vi "testaCorrente+PSuc.vi"() -> ()   [LabVIEW 2019]
uses:
  <vilib>/DAQmx/write.llb/DAQmx Write (Digital Bool 1Line 1Point).vi
  <vilib>/Analysis/5stat.llb/RMS (DBL).vi
  <vilib>/DAQmx/write.llb/DAQmx Write (Counter Frequency 1Chan 1Samp).vi
  <vilib>/DAQmx/create/channels.llb/DAQmx Create Channel (DO-Digital Output).vi
  <vilib>/DAQmx/miscellaneous.llb/DAQmx Fill In Error Info.vi
  <vilib>/DAQmx/create/channels.llb/DAQmx Create Channel (CO-Pulse Generation-Frequency).vi
  <vilib>/DAQmx/configure/timing.llb/DAQmx Timing (Implicit).vi
  <resource>/objmgr/daqmx.rc
  <vilib>/Analysis/NI_AALPro.lvlib
  <vilib>/Analysis/NI_AALBase.lvlib
panel:
  out "Array":sgl[](array[numeric])
  out "Numeric":dbl
  out "Reading":bool=TRUE
  in  "STOP":bool
  out "Erro Corrente":errorcluster
  in  "Tab Control":T1(tab)
  out "GE Comp S [bar]":dbl
  out "GE Valv S [bar]":dbl
  out "Grafico Pressão":T2(graph)
  in  "Ativar Ventilador?":bool=TRUE
  out "Descarga [bar]":dbl
  out "Sucção [bar]":dbl
  out "Corrente RMS [A]":dbl
  out "Grafico Corrente":dbl(graph)
  out "Posição Atual da Válvula de Descarga":dbl format="%#_9f"
  out "Intermed [bar]":dbl
  in  "Frequência PWM [Hz]":dbl=2.0 min=1e-12
  out "G Pressão de Descarga":cluster{"Descarga [bar]":dbl}(graph)
  out "G Pressão de Sucção":cluster{"Sucção [bar]":dbl}(graph)
  out "G Corrente RMS":dbl(graph)
  out "G Pressão Intermed":dbl(graph)
  out "Error Out":errorcluster
  in  "Limpar Gráficos":bool
  out "Tempo de Ensaio":string
  in  "Ativar Compressor?":bool
  out "Erro Valv. Sucção":errorcluster
  out "Erro Pressão":errorcluster
  # "Pressão"
  # "Temperatura"
  # "Corrente"
  # "Vazão"
  # "Vibração"
  # "Controle Manual"
  # "Controle Aplicado"
  # "PID"
  # "Ranges"
  # "Arquivos"
  # "Resistência"
  # "Identificação de sistemas"
  # "Erros"
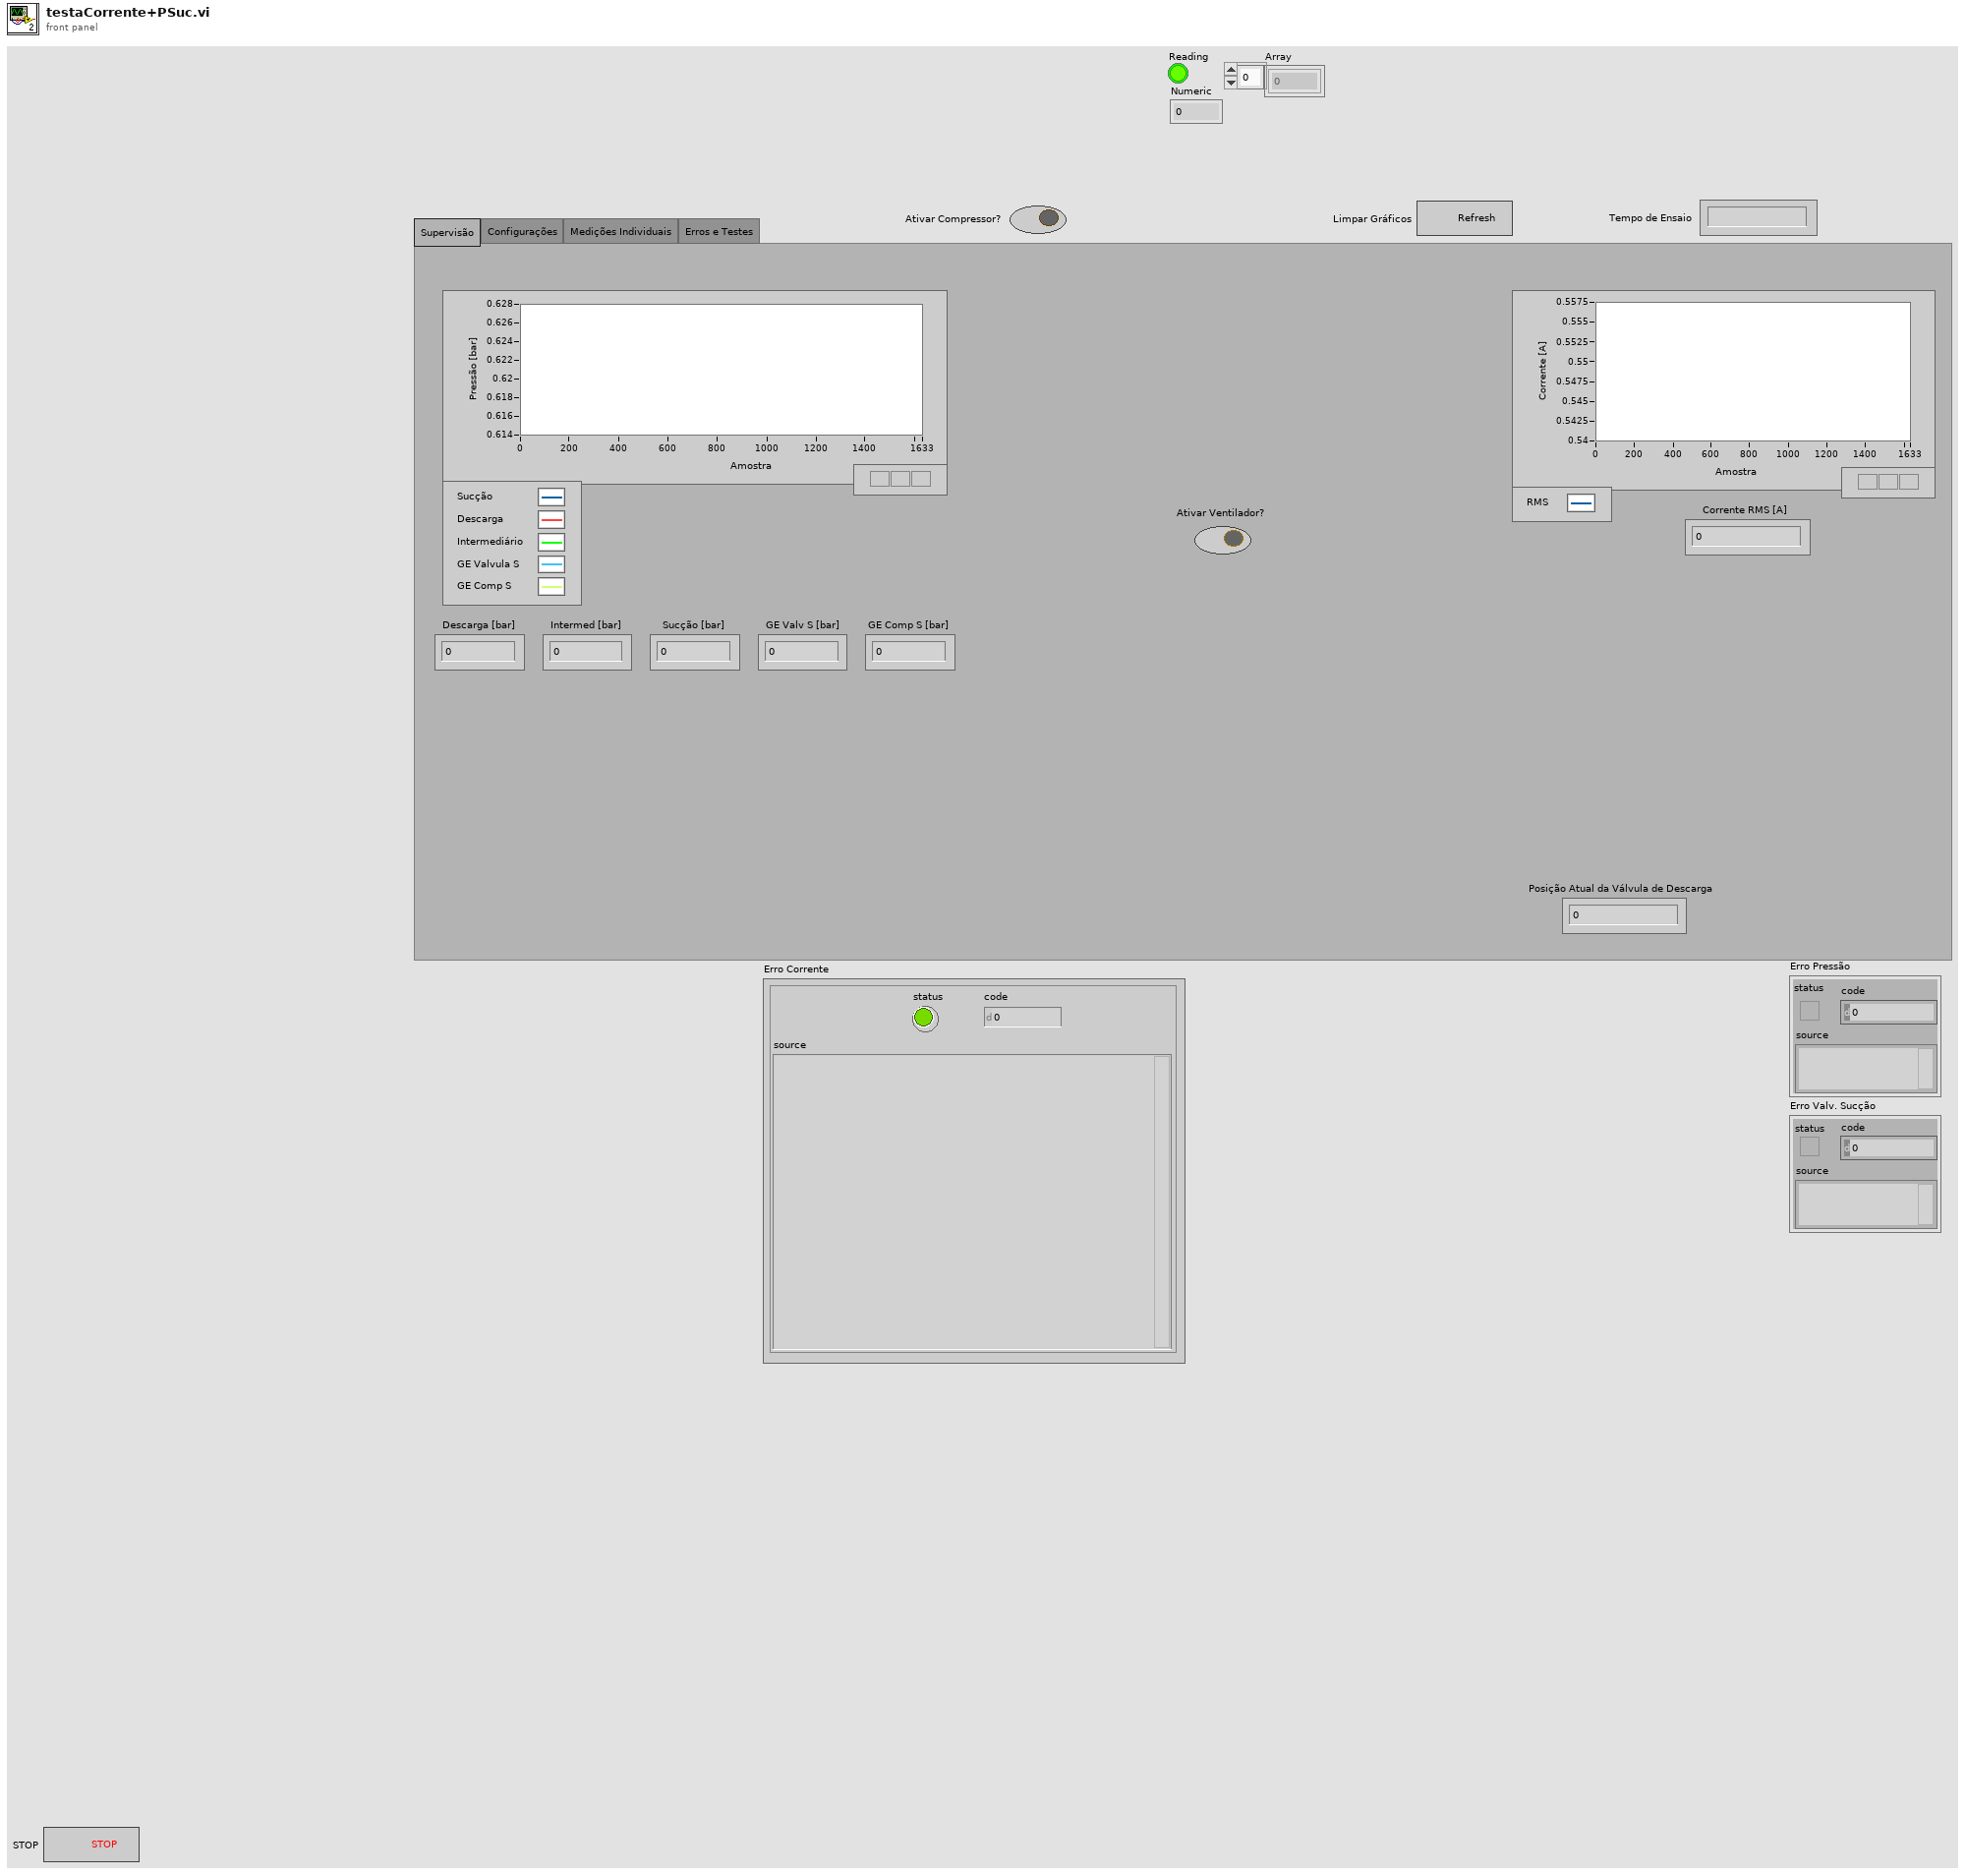
[diagram p1: front panel]
types:
  T1 = enum32{"Supervisão", "Configurações", "Medições Individuais", "Erros e Testes"}
  T2 = cluster{"Sucção [bar]":dbl, "Descarga [bar]":dbl, "Intermed [bar]":dbl, "GE Valv S [bar]":dbl, "GE Comp S [bar]":dbl}
  T3 = cluster{"Sucção [bar]":dbl, "Descarga [bar]":dbl, "Intermed [bar]":dbl, "GE Valv S [bar]":dbl, "GE Comp S [bar]":dbl}[]
  T4 = cluster{"protocolStackName":string, "interfaceName":string, "portName":string, "baudrate":u32, "timeout":u32}
  T5 = cluster{"deviceName":string, "NodeID":u8, "velocity profile":cluster{"profileAcceleration":u32, "profileDeceleration":u32}}
  T6 = typedef "xobjhandle.ctl" = u32
  T7 = cluster{"Task Analógico":refnum<k21>, "Task Clock":refnum<k21>, "Task Acionador":refnum<k21>, "Task Trigger":tag}
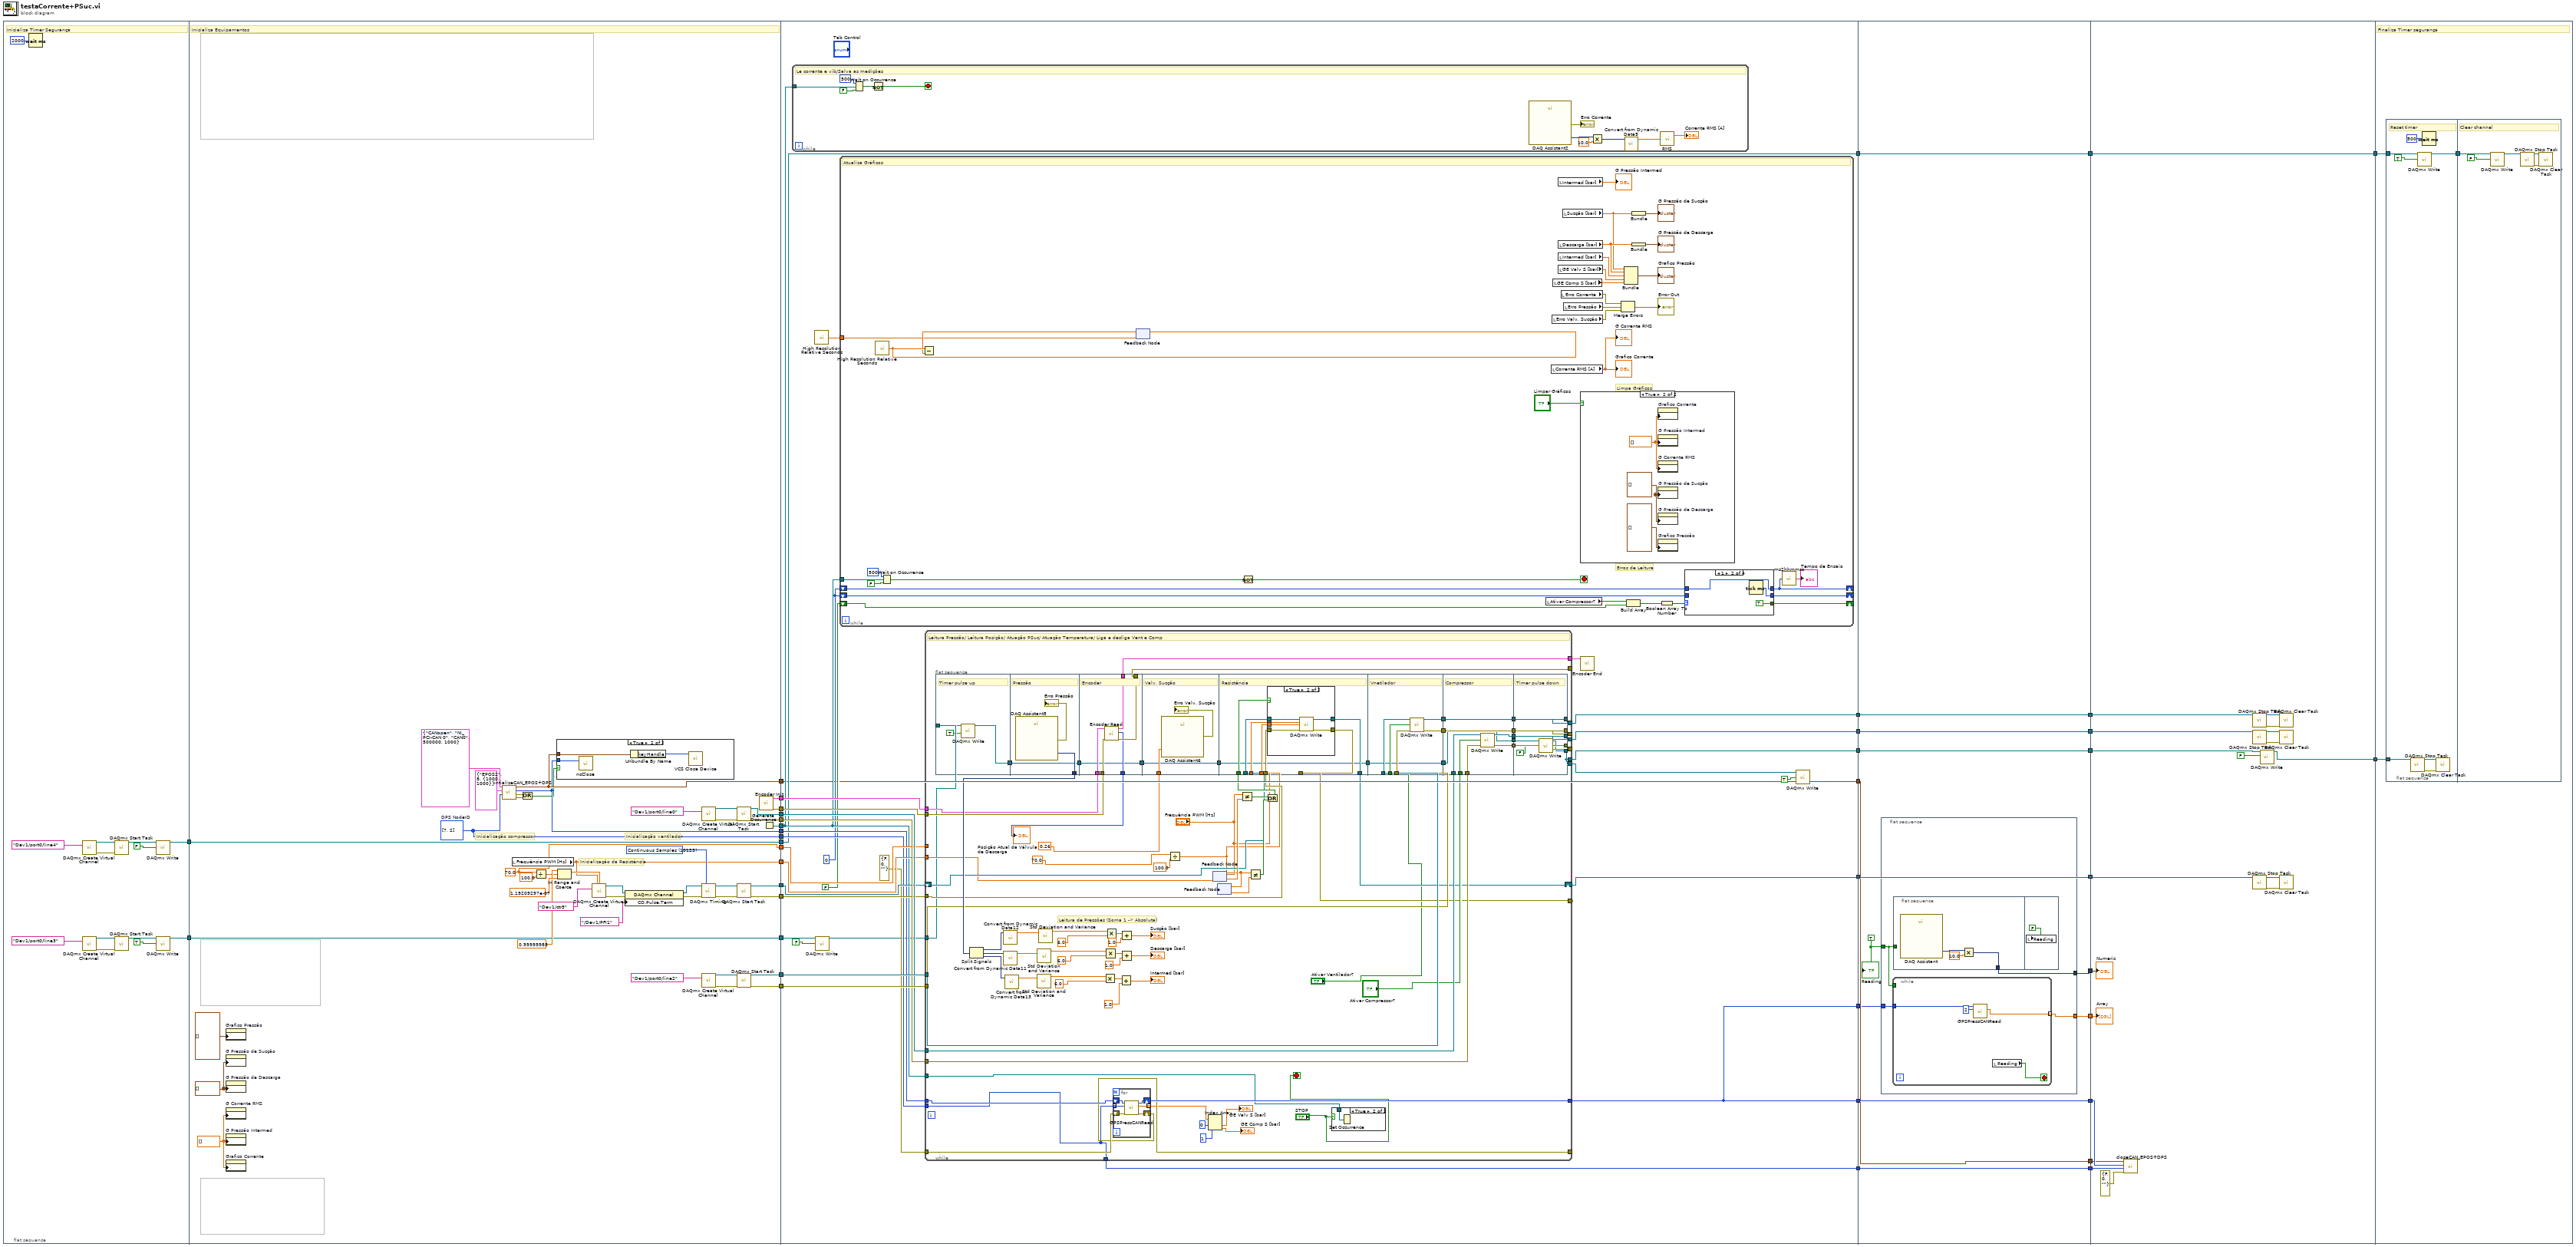
[diagram p0: block diagram]
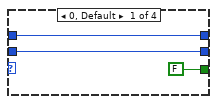
[diagram p5: hidden frame]
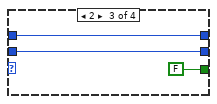
[diagram p6: hidden frame]
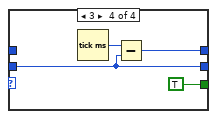
[diagram p7: hidden frame]
diagram:
  n1 = flat-sequence {
    tunnel: [w44] -> w39
    tunnel: [w43] -> w38
    tunnel: [w95] -> w27
    tunnel: [w64] -> w28
    tunnel: [w94] -> w29
    tunnel: [w96] -> w30
    tunnel: [w93] -> w31
    tunnel: [w85] -> w32
    tunnel: [w84] -> w33
    tunnel: [w83] -> w34
    tunnel: [w82] -> w35
    tunnel: [w53] -> w36
    tunnel: [w67] -> w37
    tunnel: [w65] -> w26
    tunnel: [w63] -> w25
    tunnel: [w62] -> w24
    tunnel: [w55] -> w23
    tunnel: w39 -> [w55]
    tunnel: [w54] -> w22
    tunnel: w38 -> [w54]
    tunnel: w37 -> [w121]
    tunnel: w36 -> [w122]
    tunnel: w35 -> [w130]
    tunnel: w34 -> [w129]
    tunnel: w33 -> [w127]
    tunnel: w32 -> [w128]
    tunnel: w31 -> [w125]
    tunnel: w30 -> [w124]
    tunnel: w29 -> [w123]
    tunnel: w28 -> [w101]
    tunnel: w27 -> [w126]
    tunnel: w26 -> [w118]
    tunnel: w25 -> [w116]
    tunnel: w24 -> [w117]
    tunnel: w23 -> [w114]
    tunnel: [w114] -> w19
    tunnel: w22 -> [w112]
    tunnel: [w108] -> w17
    tunnel: [w107] -> w15
    tunnel: [w106] -> w13
    tunnel: [w105] -> w11
    tunnel: [w102] -> w8
    tunnel: [w100] -> w6
    tunnel: [w101] -> w4
    tunnel: [w100] -> w3
    tunnel: w19 -> [w340]
    tunnel: [w340] -> w18
    tunnel: w17 -> [w339]
    tunnel: [w339] -> w16
    tunnel: w15 -> [w338]
    tunnel: [w338] -> w14
    tunnel: w13 -> [w337]
    tunnel: [w337] -> w12
    tunnel: w11 -> [w336]
    tunnel: [w336] -> w10
    tunnel: [w335] -> w9
    tunnel: w8 -> [w335]
    tunnel: [w334] -> w7
    tunnel: w6 -> [w334]
    tunnel: [w333] -> w5
    tunnel: w4 -> [w333]
    tunnel: w3 -> [w332]
    tunnel: [w331] -> w2
    tunnel: [w329] -> w1
    tunnel: w18 -> [w371]
    tunnel: [w371] -> w21
    tunnel: [w359] -> w20
    tunnel: w16 -> [w364]
    tunnel: w14 -> [w362]
    tunnel: w12 -> [w361]
    tunnel: w10 -> [w360]
    tunnel: w9 -> [w357]
    tunnel: w7 -> [w356]
    tunnel: w5 -> [w355]
    tunnel: w2 -> [w354]
    tunnel: w1 -> [w353]
    tunnel: w21 -> [w373]
    tunnel: w20 -> [w374]
    frame #0 {
      # "Inicializa Timer Segurança"
      n2 = Wait (ms)(milliseconds to wait=u32 2000) -> ()  [unwired: 1 out]
      n3 = call-poly <vilib>:"DAQmx Create Virtual Channel.vi"("lines"=tag "Dev1/port0/line4") -> ("task out"=w49:refnum<k21>, "error out"=w50:errorcluster)  [unwired: 13 in]
      n4 = call-poly <vilib>:"DAQmx Create Virtual Channel.vi"("lines"=tag "Dev1/port0/line3") -> ("task out"=w47:refnum<k21>, "error out"=w46:errorcluster)  [unwired: 13 in]
      n5 = call <vilib>:"DAQmx Start Task.vi"("task/channels in"=w49, "error in"=w50) -> ("task out"=w48:refnum<k21>)  [unwired: 12 in, 1 out]
      n6 = call <vilib>:"DAQmx Start Task.vi"("task/channels in"=w47, "error in"=w46) -> ("task out"=w45:refnum<k21>)  [unwired: 12 in, 1 out]
      n7 = call-poly <vilib>:"DAQmx Write.vi"("task/channels in"=w48, "data"=FALSE) -> ("task out"=w44:refnum<k21>)  [unwired: 11 in, 2 out]
      n8 = call-poly <vilib>:"DAQmx Write.vi"("task/channels in"=w45, "data"=TRUE) -> ("task out"=w43:refnum<k21>)  [unwired: 11 in, 2 out]
    }
    frame #1 {
      w53 = 70.0 ("y")
      w62 = u32[] [7, 2]  # DPS NodeID
      w72 = 10123 items=["Finite Samples"=10178, "Continuous Samples"=10123, "Hardware Timed Single Point"=12522] ("sample mode")
      w86 = dbl[] [] ("History Data")
      w66 = cluster{"Sucção [bar]":dbl}[] [] ("History Data")
      # "Inicialização ventilador"
      # "Inicialização compressor"
      # "Inicialização da Resistência"
      # "Inicializa Equipamentos"
      n9 = property on="Grafico Pressão" class="WFChart (strict)"("History Data"=T3 []) -> ()  [unwired: 2 in, 2 out]
      n10 = property on="G Pressão de Sucção" class="WFChart (strict)"("History Data"=w66) -> ()  [unwired: 2 in, 2 out]
      n11 = property on="G Pressão de Descarga" class="WFChart (strict)"("History Data"=w66) -> ()  [unwired: 2 in, 2 out]
      n12 = property on="G Corrente RMS" class="WFChart (strict)"("History Data"=w86) -> ()  [unwired: 2 in, 2 out]
      n13 = property on="G Pressão Intermed" class="WFChart (strict)"("History Data"=w86) -> ()  [unwired: 2 in, 2 out]
      n14 = property on="Grafico Corrente" class="WFChart (strict)"("History Data"=w86) -> ()  [unwired: 2 in, 2 out]
      n15 = call "intializeCAN_EPOS+DPS.vi"("DPS NodeID"=w62, "EPOS Settings"=T5 {"deviceName"="EPOS2", "NodeID"=8, "velocity profile"={"profileAcceleration"=1000, "profileDeceleration"=1000}}, "CAN Settings"=T4 {"protocolStackName"="CANopen", "interfaceName"="NI_PCI-CAN 0", "portName"="CAN0", "baudrate"=500000, "timeout"=1000}) -> ("DPS error out"=w58:errorcluster, "EPOS error out"=w57:errorcluster, "ObjHandle out"=w63:T6, "axis out"=w64:cluster{"keyHandle":u32, "nodeId":u16})  [unwired: 1 in]
      n16 = local read "Frequência PWM [Hz]"() -> (w67:dbl)
      n17 = Or(x=w57, y=w58) -> (x .or. y?=w59:bool)
      n18 = Divide(x=w53, y=100.0) -> (x/y=w76:dbl)
      n19 = case shown="True" w59 {
        tunnel: w64 -> [_ w98]
        tunnel: w63 -> [_ w97]
        frame False {
        }
        frame True {
          n20 = call <vilib>:"ncClose.vi"("ObjHandle in"=w97) -> ()  [unwired: 2 in, 1 out]
          n21 = Unbundle By Name(w98) -> ("keyHandle"=w99:u32)
          n22 = call <instrlib>:"VCS Close Device.vi"("keyHandle in"=w99) -> ()  [unwired: 10 in, 1 out]
        }
      }
      n23 = In Range and Coerce(upper limit=0.99999988 ("output high"), x=w76, lower limit=1.19209297e-07 ("output low")) -> (coerced(x)=w81:dbl)  [unwired: 1 out]
      n24 = call-poly <vilib>:"DAQmx Create Virtual Channel.vi"("frequency"=w67, "duty cycle"=w81, "counter"=tag "Dev1/ctr3") -> ("task out"=w69:refnum<k21>, "error out"=w68:errorcluster)  [unwired: 11 in]
      n25 = property class="DAQmx Channel"(reference=w69, error in=w68, "CO.Pulse.Term"=tag "/Dev1/PFI1") -> (reference out=w74:refnum<k21>, error out=w70:errorcluster)
      n26 = call-poly <vilib>:"DAQmx Timing.vi"("task/channels in"=w74, "sample mode"=w72, "error in"=w70) -> ("task out"=w73:refnum<k21>, "error out"=w75:errorcluster)  [unwired: 11 in]
      n27 = call-poly <vilib>:"DAQmx Create Virtual Channel.vi"("lines"=tag "Dev1/port0/line0") -> ("task out"=w92:refnum<k21>, "error out"=w91:errorcluster)  [unwired: 13 in]
      n28 = call-poly <vilib>:"DAQmx Create Virtual Channel.vi"("lines"=tag "Dev1/port0/line2") -> ("task out"=w89:refnum<k21>, "error out"=w88:errorcluster)  [unwired: 13 in]
      n29 = call <vilib>:"DAQmx Start Task.vi"("task/channels in"=w92, "error in"=w91) -> ("task out"=w95:refnum<k21>, "error out"=w93:errorcluster)  [unwired: 12 in]
      n30 = call <vilib>:"DAQmx Start Task.vi"("task/channels in"=w73, "error in"=w75) -> ("task out"=w94:refnum<k21>, "error out"=w96:errorcluster)  [unwired: 12 in]
      n31 = call <vilib>:"DAQmx Start Task.vi"("task/channels in"=w89, "error in"=w88) -> ("task out"=w85:refnum<k21>, "error out"=w84:errorcluster)  [unwired: 12 in]
      n32 = call "Encoder Init.vi"() -> ("error out"=w82:errorcluster, "Task Out"=w83:T7)  [unwired: 10 in]
      n33 = Generate Occurrence() -> (w65:refnum<k4>)
    }
    frame #2 {
      w109 = u32 0 ("millisecond timer value")
      n34 = while {
        tunnel: w118 -> [w318]
        stop <- w319 stop-if-true
        # "Le corrente e vib/Salva as medições"
        n35 = Wait on Occurrence(1:FALSE ("ignore previous (T)"), 2:w318, 3:500 ("ms timeout (-1)")) -> (0:w322:bool)
        n36 = Not(x=w322) -> (.not. x?=w319:bool)
        n37 = call "DAQ Assistant2"() -> ("data"=w323:dynamicdata, "error out"=→"Erro Corrente":errorcluster)  [unwired: 17 in, 1 out]
        n38 = Multiply(x=w323, y=10.0) -> (x*y=w325:dynamicdata)
        n39 = call "Convert from Dynamic Data5"("Dynamic Data Type"=w325) -> ("Array"=w326:dbl[])  [unwired: 3 in]
        n40 = call-poly <vilib>:"RMS.vi"("X"=w326) -> ("rms value"=→"Corrente RMS [A]":dbl)  [unwired: 1 out]
      }
      n41 = call <vilib>:"High Resolution Relative Seconds.vi"() -> ("relative seconds"=w120:dbl)
      n42 = call-poly <vilib>:"DAQmx Write.vi"("task/channels in"=w112, "data"=FALSE) -> ("task out"=w111:refnum<k21>)  [unwired: 11 in, 2 out]
      n43 = while {
        tunnel: w120 -> [w299]
        tunnel: w118 -> [w288]
        shift-right: [w274] -> _
        shift-left: FALSE -> [w279]
        shift-right: [w273] -> _
        shift-left: w109 -> [w276]
        shift-right: [w272] -> _
        shift-left: w109 -> [w275]
        stop <- w287 stop-if-true
        # "Erros de Leitura"
        # "Limpa Gráficos"
        # "Atualiza Gráficos"
        n44 = call <vilib>:"High Resolution Relative Seconds.vi"() -> ("relative seconds"=w301:dbl)
        n45 = Wait on Occurrence(1:FALSE ("ignore previous (T)"), 2:w288, 3:500 ("ms timeout (-1)")) -> (0:w290:bool)
        n46 = feedback #1(w299) -> (w300:dbl)
        n47 = Subtract(x=w301, y=w300) -> ()  [unwired: 1 out]
        n48 = feedback-in #1(w301) -> ()
        n49 = Not(x=w290) -> (.not. x?=w287:bool)
        n50 = local read "Ativar Compressor?"() -> (w280:bool)
        n51 = local read "Corrente RMS [A]"() -> (→"Grafico Corrente" →"G Corrente RMS":dbl)
        n52 = local read "Erro Valv. Sucção"() -> (w269:errorcluster)
        n53 = local read "GE Comp S [bar]"() -> (w281:dbl)
        n54 = local read "Intermed [bar]"() -> (→"G Pressão Intermed":dbl)
        n55 = local read "Descarga [bar]"() -> (w294:dbl)
        n56 = local read "Intermed [bar]"() -> (w291:dbl)
        n57 = local read "GE Valv S [bar]"() -> (w283:dbl)
        n58 = local read "Erro Corrente"() -> (w284:errorcluster)
        n59 = local read "Sucção [bar]"() -> (w282:dbl)
        n60 = local read "Erro Pressão"() -> (w270:errorcluster)
        n61 = case shown="True" "Limpar Gráficos" {
          frame False {
          }
          frame True {
            w317 = dbl[] [] ("History Data")
            w316 = cluster{"Sucção [bar]":dbl}[] [] ("History Data")
            n62 = property on="Grafico Corrente" class="WFChart (strict)"("History Data"=w317) -> ()  [unwired: 2 in, 2 out]
            n63 = property on="G Pressão Intermed" class="WFChart (strict)"("History Data"=w317) -> ()  [unwired: 2 in, 2 out]
            n64 = property on="G Corrente RMS" class="WFChart (strict)"("History Data"=w317) -> ()  [unwired: 2 in, 2 out]
            n65 = property on="G Pressão de Sucção" class="WFChart (strict)"("History Data"=w316) -> ()  [unwired: 2 in, 2 out]
            n66 = property on="G Pressão de Descarga" class="WFChart (strict)"("History Data"=w316) -> ()  [unwired: 2 in, 2 out]
            n67 = property on="Grafico Pressão" class="WFChart (strict)"("History Data"=T3 []) -> ()  [unwired: 2 in, 2 out]
          }
        }
        n68 = Merge Errors(w284, w270, w269) -> (→"Error Out":errorcluster)
        n69 = Bundle("Sucção [bar]"=w282, "Descarga [bar]"=w294, "Intermed [bar]"=w291, "GE Valv S [bar]"=w283, "GE Comp S [bar]"=w281) -> (→"Grafico Pressão":T2)  [unwired: 1 in]
        n70 = Build Array(w280, w279) -> (w278:bool[])
        n71 = Bundle("Sucção [bar]"=w282) -> (→"G Pressão de Sucção":cluster{"Sucção [bar]":dbl})  [unwired: 1 in]
        n72 = Bundle("Descarga [bar]"=w294) -> (→"G Pressão de Descarga":cluster{"Descarga [bar]":dbl})  [unwired: 1 in]
        n73 = Boolean Array To Number(Boolean array=w278) -> (number=w277:u32)
        n74 = case shown="1" w277 {
          tunnel: w276 -> [w302 _ w309 w312]
          tunnel: w275 -> [w303 w305 w310 _]
          tunnel: [w303 w305 w310 w313] -> w272
          tunnel: [FALSE TRUE FALSE TRUE] -> w274
          tunnel: [w302 w307 w309 w312] -> w273
          frame 0, Default {
          }
          frame 1 {
            n75 = Tick Count (ms)() -> (millisecond timer value=w307:u32)
          }
          frame 2 {
          }
          frame 3 {
            n76 = Tick Count (ms)() -> (millisecond timer value=w314:u32)
            n77 = Subtract(x=w314, y=w312) -> (x-y=w313:u32)
          }
        }
        n78 = call "ms2hhmmss.vi"("ms"=w272) -> ("hh:mm:ss"=→"Tempo de Ensaio":string)
      }
      n79 = while {
        tunnel: [w181] -> w106
        tunnel: [w180] -> _
        tunnel: [w174] -> w105
        tunnel: [w173] -> _
        tunnel: [w185] -> _
        tunnel: w130 -> [w187]
        tunnel: w129 -> [w186]
        tunnel: w128 -> [w183]
        tunnel: w127 -> [w182]
        tunnel: w126 -> [w177]
        tunnel: w125 -> [w175]
        tunnel: w124 -> [w167]
        shift-right: [w166] -> w107
        shift-left: w123 -> [w165]
        tunnel: [w164] -> _
        tunnel: w122 -> [_]
        tunnel: w121 -> [w163]
        tunnel: w118 -> [w132]
        tunnel: [w159] -> w119
        tunnel: w117 -> [w153]
        tunnel: w116 -> [w157]
        tunnel: errorcluster {"status"=FALSE, "code"=0, "source"=""} ("error out") -> [w156]
        tunnel: [w155] -> w100
        tunnel: [w154] -> _
        tunnel: [w153] -> w102
        tunnel: w111 -> [w147]
        tunnel: [w131] -> w108
        tunnel: [w131] -> w104
        stop <- "STOP" stop-if-true
        # "Leitura de Pressões (Soma 1 -> Absoluta)"
        # "Leitura Pressão/ Leitura Posição/ Atuação PSuc/ Atuação Temperatura/ Liga e desliga Vent e Comp"
        n80 = flat-sequence {
          tunnel: w147 -> [w218]
          tunnel: [w217] -> w142
          tunnel: [w222] -> w188
          tunnel: w142 -> [w220]
          tunnel: [w220] -> w141
          tunnel: w187 -> [w228]
          tunnel: w186 -> [w227]
          tunnel: [w226] -> w185
          tunnel: [w225] -> w184
          tunnel: [w224] -> w159
          tunnel: w141 -> [w223]
          tunnel: [w223] -> w140
          tunnel: 0.26 ("y") -> [w231]
          tunnel: w140 -> [w229]
          tunnel: [w229] -> w139
          tunnel: w168 -> [w233]
          tunnel: "Frequência PWM [Hz]" -> [w239]
          tunnel: w160 -> [w238]
          tunnel: w165 -> [w237]
          tunnel: w167 -> [w236]
          tunnel: [w235] -> w166
          tunnel: [w234] -> w164
          tunnel: w139 -> [w232]
          tunnel: [w232] -> w138
          tunnel: w183 -> [w253]
          tunnel: w182 -> [w252]
          tunnel: [w251] -> w179
          tunnel: [w250] -> w178
          tunnel: "Ativar Ventilador?" -> [w249]
          tunnel: w138 -> [w248]
          tunnel: [w248] -> w137
          tunnel: w179 -> [w261]
          tunnel: w178 -> [w260]
          tunnel: w177 -> [w259]
          tunnel: "Ativar Compressor?" -> [w258]
          tunnel: w175 -> [w257]
          tunnel: [w261] -> w146
          tunnel: [w260] -> w145
          tunnel: [w256] -> w144
          tunnel: [w255] -> w143
          tunnel: w137 -> [w254]
          tunnel: [w254] -> w136
          tunnel: [w265] -> w173
          tunnel: [w266] -> w174
          tunnel: [w267] -> w180
          tunnel: [w268] -> w181
          tunnel: w146 -> [w268]
          tunnel: w145 -> [w267]
          tunnel: w144 -> [w266]
          tunnel: w143 -> [w265]
          tunnel: w136 -> [w263]
          tunnel: [w262] -> w131
          frame #0 {
            # "Timer pulse up"
            n81 = call-poly <vilib>:"DAQmx Write.vi"("task/channels in"=w218, "data"=TRUE) -> ("task out"=w217:refnum<k21>)  [unwired: 11 in, 2 out]
          }
          frame #1 {
            # "Pressão"
            n82 = call "DAQ Assistant5"() -> ("data"=w222:dynamicdata, "error out"=→"Erro Pressão":errorcluster)  [unwired: 17 in, 1 out]
          }
          frame #2 {
            # "Encoder"
            n83 = call "Encoder Read.vi"("error in (no error)"=w228, "Task In"=w227) -> ("error out"=w226:errorcluster, "Posição"=w225:i32, "Task Out"=w224:T7)  [unwired: 7 in]
          }
          frame #3 {
            # "Valv. Sucção"
            n84 = call "DAQ Assistant6"("data"=w231) -> ("error out"=→"Erro Valv. Sucção":errorcluster)  [unwired: 17 in, 1 out]
          }
          frame #4 {
            # "Resistência"
            n85 = case shown="True" w233 {
              tunnel: w239 -> [_ w247]
              tunnel: w238 -> [_ w246]
              tunnel: w237 -> [w241 w245]
              tunnel: w236 -> [w240 w244]
              tunnel: [w241 w243] -> w235
              tunnel: [w240 w242] -> w234
              frame False {
              }
              frame True {
                n86 = call-poly <vilib>:"DAQmx Write.vi"("task/channels in"=w245, "frequency"=w247, "duty cycle"=w246, "error in"=w244) -> ("task out"=w243:refnum<k21>, "error out"=w242:errorcluster)  [unwired: 9 in, 1 out]
              }
            }
          }
          frame #5 {
            # "Vnetilador"
            n87 = call-poly <vilib>:"DAQmx Write.vi"("task/channels in"=w253, "data"=w249, "error in"=w252) -> ("task out"=w251:refnum<k21>, "error out"=w250:errorcluster)  [unwired: 10 in, 1 out]
          }
          frame #6 {
            # "Compressor"
            n88 = call-poly <vilib>:"DAQmx Write.vi"("task/channels in"=w259, "data"=w258, "error in"=w257) -> ("task out"=w256:refnum<k21>, "error out"=w255:errorcluster)  [unwired: 10 in, 1 out]
          }
          frame #7 {
            # "Timer pulse down"
            n89 = call-poly <vilib>:"DAQmx Write.vi"("task/channels in"=w263, "data"=FALSE) -> ("task out"=w262:refnum<k21>)  [unwired: 11 in, 2 out]
          }
        }
        n90 = Split Signals(w188) -> (w201:dynamicdata, w202:dynamicdata, w205:dynamicdata)  [unwired: 3 in]
        n91 = call "Convert from Dynamic Data12"("Dynamic Data Type"=w201) -> ("Array"=w198:dbl[])  [unwired: 3 in]
        n92 = call "Convert from Dynamic Data11"("Dynamic Data Type"=w202) -> ("Array"=w199:dbl[])  [unwired: 3 in]
        n93 = call "Convert from Dynamic Data13"("Dynamic Data Type"=w205) -> ("Array"=w206:dbl[])  [unwired: 3 in]
        n94 = call <vilib>:"Std Deviation and Variance.vi"("X"=w206) -> ("mean"=w207:dbl)  [unwired: 1 in, 2 out]
        n95 = call <vilib>:"Std Deviation and Variance.vi"("X"=w199) -> ("mean"=w193:dbl)  [unwired: 1 in, 2 out]
        n96 = call <vilib>:"Std Deviation and Variance.vi"("X"=w198) -> ("mean"=w191:dbl)  [unwired: 1 in, 2 out]
        n97 = Multiply(x=w207, y=6.0) -> (x*y=w208:dbl)
        n98 = Multiply(x=w193, y=6.0) -> (x*y=w196:dbl)
        n99 = Multiply(x=w191, y=6.0) -> (x*y=w197:dbl)
        n100 = for {
          tunnel: [w214] -> w149 mode=indexing
          shift-right: [w211] -> w154
          shift-left: w156 -> [w212]
          shift-right: [w213] -> w155
          shift-left: w157 -> [w215]
          tunnel: w153 -> [w210] mode=indexing
          n101 = call "GPSPressCANRead.vi"("Error In"=w212, "NodeID"=w210, "ObjHandle In"=w215) -> ("Error Out"=w211:errorcluster, "Pressure"=w214:sgl, "ObjHandle Out"=w213:u32)  [unwired: 6 in]
        }
        n102 = Add(x=w208, y=1.0) -> (x+y=→"Intermed [bar]":dbl)
        n103 = Add(x=w197, y=1.0) -> (x+y=→"Sucção [bar]":dbl)
        n104 = Add(x=w196, y=1.0) -> (x+y=→"Descarga [bar]":dbl)
        n105 = Divide(x=70.0 ("y"), y=100.0) -> (x/y=w160:dbl)
        n106 = Index Array(array=w149, index #1=0 ("index"), index #2=1 ("index")) -> (element #1=→"GE Valv S [bar]":sgl, element #2=→"GE Comp S [bar]":sgl)
        n107 = feedback #2(w163) -> (w172:dbl)
        n108 = feedback-in #2("Frequência PWM [Hz]") -> ()
        n109 = feedback #3() -> (w171:dbl)  [unwired: 1 in]
        n110 = feedback-in #3(w160) -> ()
        n111 = Not Equal?(x="Frequência PWM [Hz]", y=w172) -> (x != y?=w170:bool)
        n112 = Not Equal?(x=w160, y=w171) -> (x != y?=w169:bool)
        n113 = Or(x=w170, y=w169) -> (x .or. y?=w168:bool)
        n114 = case shown="True" "STOP" {
          tunnel: w132 -> [_ w216]
          frame False {
          }
          frame True {
            n115 = Set Occurrence(w216) -> ()
          }
        }
        "Posição Atual da Válvula de Descarga" <- w184
      }
      n116 = call "Encoder End.vi"("Task Out"=w119) -> ()  [unwired: 10 in, 1 out]
      n117 = call-poly <vilib>:"DAQmx Write.vi"("task/channels in"=w104, "data"=TRUE) -> ()  [unwired: 11 in, 3 out]
    }
    frame #3 {
      w330 = TRUE
      n118 = flat-sequence {
        tunnel: w332 -> [w344]
        tunnel: [w343] -> w331
        tunnel: w330 -> [w342]
        tunnel: [w341] -> w329
        frame #0 {
          n119 = while {
            tunnel: w344 -> [w352]
            tunnel: [w350] -> w341 mode=indexing
            tunnel: w342 -> [_]
            stop <- w349 stop-if-true
            n120 = call "GPSPressCANRead.vi"("NodeID"=u8 2, "ObjHandle In"=w352) -> ("Pressure"=w350:sgl)  [unwired: 7 in, 2 out]
            n121 = local read "Reading"() -> (w349:bool)
          }
          n122 = flat-sequence {
            tunnel: [w345] -> w343
            tunnel: w342 -> [_]
            frame #0 {
              n123 = call "DAQ Assistant"() -> ("data"=w346:dynamicdata)  [unwired: 17 in, 2 out]
              n124 = Multiply(x=w346, y=10.0) -> (x*y=w345:dynamicdata)
            }
            frame #1 {
              n125 = local write "Reading"(FALSE) -> ()
            }
          }
        }
      }
      "Reading" <- w330
    }
    frame #4 {
      n126 = call "closeCAN_EPOS+DPS.vi"("error in"=errorcluster {"status"=FALSE, "code"=0, "source"=""} ("error out"), "DPS NodeID"=w357, "ObjHandle in"=w356, "axis in"=w355) -> ()  [unwired: 7 in, 1 out]
      n127 = call <vilib>:"DAQmx Stop Task.vi"("task/channels in"=w361) -> ("task out"=w366:refnum<k21>, "error out"=w365:errorcluster)  [unwired: 13 in]
      n128 = call <vilib>:"DAQmx Stop Task.vi"("task/channels in"=w360) -> ("task out"=w368:refnum<k21>, "error out"=w367:errorcluster)  [unwired: 13 in]
      n129 = call <vilib>:"DAQmx Stop Task.vi"("task/channels in"=w362) -> ("task out"=w369:refnum<k21>, "error out"=w370:errorcluster)  [unwired: 13 in]
      n130 = call-poly <vilib>:"DAQmx Write.vi"("task/channels in"=w364, "data"=FALSE) -> ("task out"=w359:refnum<k21>)  [unwired: 11 in, 2 out]
      n131 = call <vilib>:"DAQmx Clear Task.vi"("task in"=w366, "error in"=w365) -> ()  [unwired: 13 in, 1 out]
      n132 = call <vilib>:"DAQmx Clear Task.vi"("task in"=w368, "error in"=w367) -> ()  [unwired: 13 in, 1 out]
      n133 = call <vilib>:"DAQmx Clear Task.vi"("task in"=w369, "error in"=w370) -> ()  [unwired: 13 in, 1 out]
      "Numeric" <- w354
      "Array" <- w353
    }
    frame #5 {
      # "Finaliza Timer segurança"
      n134 = flat-sequence {
        tunnel: w374 -> [w380]
        tunnel: w373 -> [w377]
        tunnel: [w376] -> w372
        tunnel: w372 -> [w382]
        frame #0 {
          # "Reset timer"
          n135 = call <vilib>:"DAQmx Stop Task.vi"("task/channels in"=w380) -> ("task out"=w379:refnum<k21>, "error out"=w381:errorcluster)  [unwired: 13 in]
          n136 = call-poly <vilib>:"DAQmx Write.vi"("task/channels in"=w377, "data"=TRUE) -> ("task out"=w376:refnum<k21>)  [unwired: 11 in, 2 out]
          n137 = Wait (ms)(milliseconds to wait=u32 500) -> ()  [unwired: 1 out]
          n138 = call <vilib>:"DAQmx Clear Task.vi"("task in"=w379, "error in"=w381) -> ()  [unwired: 13 in, 1 out]
        }
        frame #1 {
          # "Clear channel"
          n139 = call-poly <vilib>:"DAQmx Write.vi"("task/channels in"=w382, "data"=FALSE) -> ("task out"=w383:refnum<k21>)  [unwired: 11 in, 2 out]
          n140 = call <vilib>:"DAQmx Stop Task.vi"("task/channels in"=w383) -> ("task out"=w385:refnum<k21>, "error out"=w386:errorcluster)  [unwired: 13 in]
          n141 = call <vilib>:"DAQmx Clear Task.vi"("task in"=w385, "error in"=w386) -> ()  [unwired: 13 in, 1 out]
        }
      }
    }
  }
